vi "Raman.vi"(1 "In":variant, 2 "Mode":u32(ring) items=["Open", "Close", "Begin", "End", "Get", "Set"]) -> (0 "Out":variant)   [LabVIEW 2014]
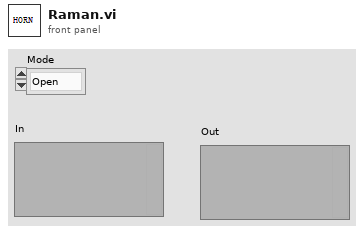
[diagram p1: front panel]
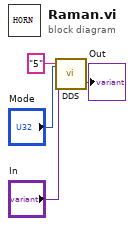
[diagram p0: block diagram]
diagram:
  n1 = call "DDS.vi"("Device"="5" ("IP"), "In"="In", "Mode"="Mode") -> ("Out"=→"Out":variant)
